vi "Manipulator Inertia Torque (Point).vi"(8 "error in (no error)":errorcluster, 9 "joint accelerations":dbl[](array[numeric]), 10 "joint positions":dbl[](array[numeric]), 11 "serial arm in":refnum<class "NI_Robotics_Serial Robot Arm.lvclass">) -> (0 "error out":errorcluster, 2 "torques":dbl[](array[numeric]), 3 "serial arm out":refnum<class "NI_Robotics_Serial Robot Arm.lvclass">)   [LabVIEW 2017, in "NI_Kinematics.lvlib"]
doc: "Calculates the joint torques that result from inertia given the joint accelerations you specify. Wire data to the <B>joint positions</B> input to determine the polymorphic instance to use or manually select the instance.\n\n<B>.m file:</B> itorque"
uses:
  <vilib>/robotics/Kinematics/NI_Kinematics.lvlib
  <vilib>/robotics/Kinematics/Robot/NI_Robotics_Serial Robot Arm.lvclass
  <vilib>/robotics/Kinematics/dyn/Inverse Dynamics (Point).vi
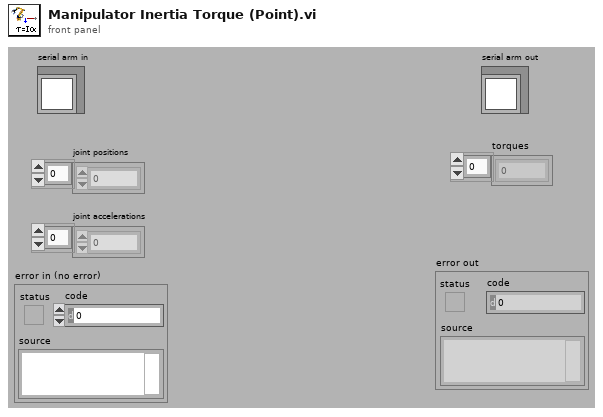
[diagram p1: front panel]
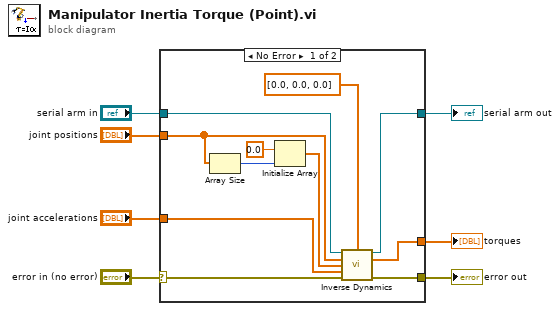
[diagram p0: block diagram]
diagram:
  n1 = case shown="No Error" "error in (no error)" {
    selector: "error in (no error)" -> [w8 w19]
    tunnel: "serial arm in" -> [w18 w20]
    tunnel: [w17 w20] -> w6
    tunnel: "joint accelerations" -> [w13 _]
    tunnel: [w11 _] -> w4
    tunnel: "joint positions" -> [w10 _]
    tunnel: [w9 w19] -> w2
    frame No Error {
      n2 = Array Size(array=w10) -> (size(s)=w16:i32)
      n3 = Initialize Array(0.0 ("element"), w16) -> (w12:dbl[])
      n4 = call-poly <vilib>:"Inverse Dynamics.vi"("serial arm in"=w18, "gravity"=dbl[] [0.0, 0.0, 0.0], "joint positions"=w10, "joint velocities"=w12, "joint accelerations"=w13, "error in (no error)"=w8) -> ("serial arm out"=w17:refnum<class "NI_Robotics_Serial Robot Arm.lvclass">, "required torques"=w11:dbl[], "error out"=w9:errorcluster)  [unwired: 7 in]
    }
    frame Error {
    }
  }
  "serial arm out" <- w6
  "torques" <- w4
  "error out" <- w2
